vi "Render EscapedVariable-Text.vi"(8 "Error In":errorcluster) -> (0 "Error Out":errorcluster)   [LabVIEW 2018, in "Tests.lvlib" / "Render.lvlib"]
uses:
  Render.lvlib
  src/Toolkit/Readers/String/String.lvclass
  D:/Users/cfield/Code/Field R&D Services/Mustache/trunk/src/Toolkit/Readers/Abstract/Abstract.lvclass
  src/Toolkit/Render/Support/Render to String.vi
  <vilib>/addons/_JKI Toolkits/Caraya/classes/Test/Test.lvclass
  <vilib>/addons/_JKI Toolkits/Caraya/classes/Assert/Assert.lvclass
  src/Toolkit/Render/Render.lvclass
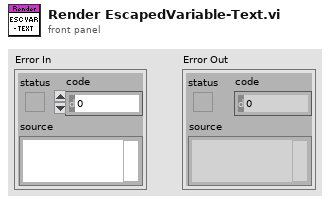
[diagram p1: front panel]
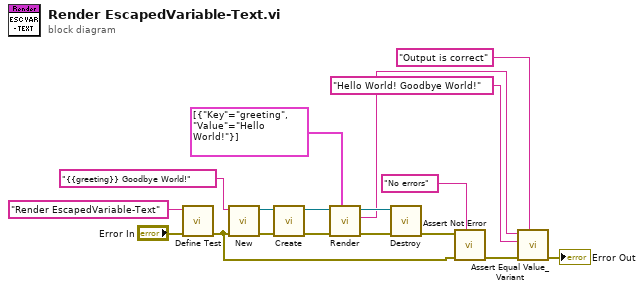
[diagram p0: block diagram]
diagram:
  n1 = call <vilib>:"Define Test.vi"("error in (no error)"="Error In", "Label (VI Title)"="Render EscapedVariable-Text") -> ("error out"=w16:errorcluster)  [unwired: 9 in]
  n2 = call "New.vi"("Error In"=w16, "String"="{{greeting}} Goodbye World!" ("format string")) -> ("Error Out"=w9:errorcluster, "String"=w10:refnum<class "String.lvclass">)  [unwired: 8 in]
  n3 = call "Create.vi"("Error In"=w9, "Reader"=w10) -> ("Error Out"=w7:errorcluster, "Render"=w8:refnum<class "Render.lvclass">)  [unwired: 8 in]
  n4 = call-poly "Render.vi"("Data"=cluster{"Key":string, "Value":string}[] [{"Key"="greeting", "Value"="Hello World!"}], "Error In"=w7, "Render In"=w8) -> ("Error Out"=w6:errorcluster, "Output"=w3:string, "Render Out"=w5:refnum<class "Render.lvclass">)  [unwired: 6 in]
  n5 = call "Destroy.vi"("Error In"=w6, "Render"=w5) -> ("Error Out"=w4:errorcluster)  [unwired: 8 in, 1 out]
  n6 = call <vilib>:"Assert Not Error.vi"("Label"="No errors", "error in (no error)"=w16, "Not Error?"=w4) -> ("error out"=w14:errorcluster)  [unwired: 8 in]
  n7 = call <vilib>:"Assert Equal Value_Variant.vi"("Label"="Output is correct", "error in (no error)"=w14, "Y"="Hello World! Goodbye World!", "X"=w3) -> ("error out"=→"Error Out":errorcluster)  [unwired: 7 in]
